vi "Displacement.vi"   [LabVIEW 2016]
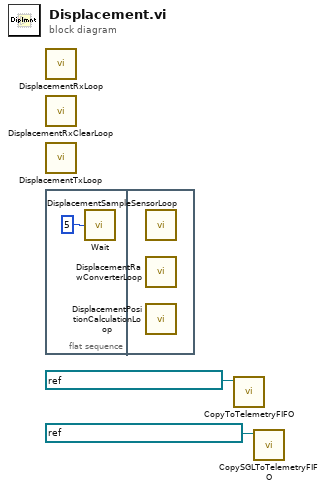
[diagram p0: block diagram]
diagram:
  n1 = call "DisplacementRxLoop.vi"() -> ()  [unwired: 12 in]
  n2 = call "DisplacementRxClearLoop.vi"() -> ()  [unwired: 12 in]
  n3 = call "DisplacementTxLoop.vi"() -> ()  [unwired: 12 in]
  n4 = flat-sequence {
    frame #0 {
      n5 = call "Wait"("Count(mSec)"=u32 5) -> ()  [unwired: 1 out]
    }
    frame #1 {
      n6 = call "DisplacementSampleSensorLoop.vi"() -> ()  [unwired: 12 in]
      n7 = call "DisplacementRawConverterLoop.vi"() -> ()  [unwired: 12 in]
      n8 = call "DisplacementPositionCalculationLoop.vi"() -> ()  [unwired: 12 in]
    }
  }
  n9 = call "CopyToTelemetryFIFO.vi"("SourceFIFO"=refnum<k21> "DisplacementTelemetryFIFO") -> ()  [unwired: 11 in]
  n10 = call "CopySGLToTelemetryFIFO.vi"("SourceFIFO"=refnum<k21> "DisplacementTelemetrySGLFIFO") -> ()  [unwired: 11 in]
